vi "SiPM_Data_Analysis.vi"() -> ()   [LabVIEW 2019]
uses:
  <vilib>/Utility/tdmsutil.llb/fileViewerConfigData.ctl
  Data_Analysis_subvis/ESA_Data_Analysis_Global_VIs.vi
panel:
  in  "Detailed":bool
  out "Indicator":bool
  in  "Listbox":i32[](listbox) caption="SiPM_laser_tests_10x.tdms"
  in  "Data tab":enum32{"Raw", "Filtered", "Properties"}(tab)
  in  "Nb of Samples as Offset":i32=50
  in  "Display sel":bool
  out "SiPM Waveform":waveform(dbl)[](graph)
  in  "Nb of Samples to Display":i32=50
  in  "Tab Sel":T1(radio)
  out "Table":string[][](table)
  in  "Stop Button":bool
  in  "Open Button":bool
  out "Nb of Channels in Group":i32
  out "group names":string[](array[string])
  out "tdms file out":refnum<k34>
  in  "File contents":string[](tree)
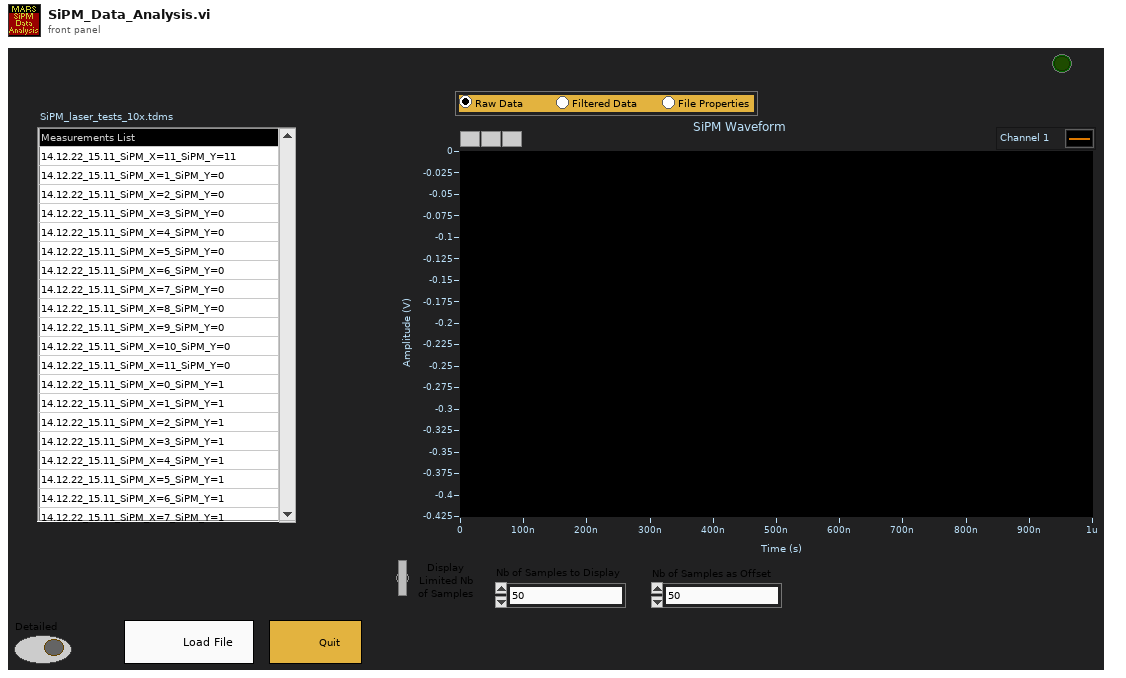
[diagram p1: front panel]
types:
  T1 = enum32{"Radio Selection 1", "Radio Selection 2", "Radio Selection 3"}
  T2 = typedef "fileViewerConfigData.ctl" = cluster{"Show all (table)":bool, "Show all (graph)":bool, "limit (table)":u64, "limit (graph)":u64, "no show":bool, "start (table)":u64, "start (graph)":u64}
  T3 = enum16{"open", "open or create", "create or replace", "create", "open (read-only)"}
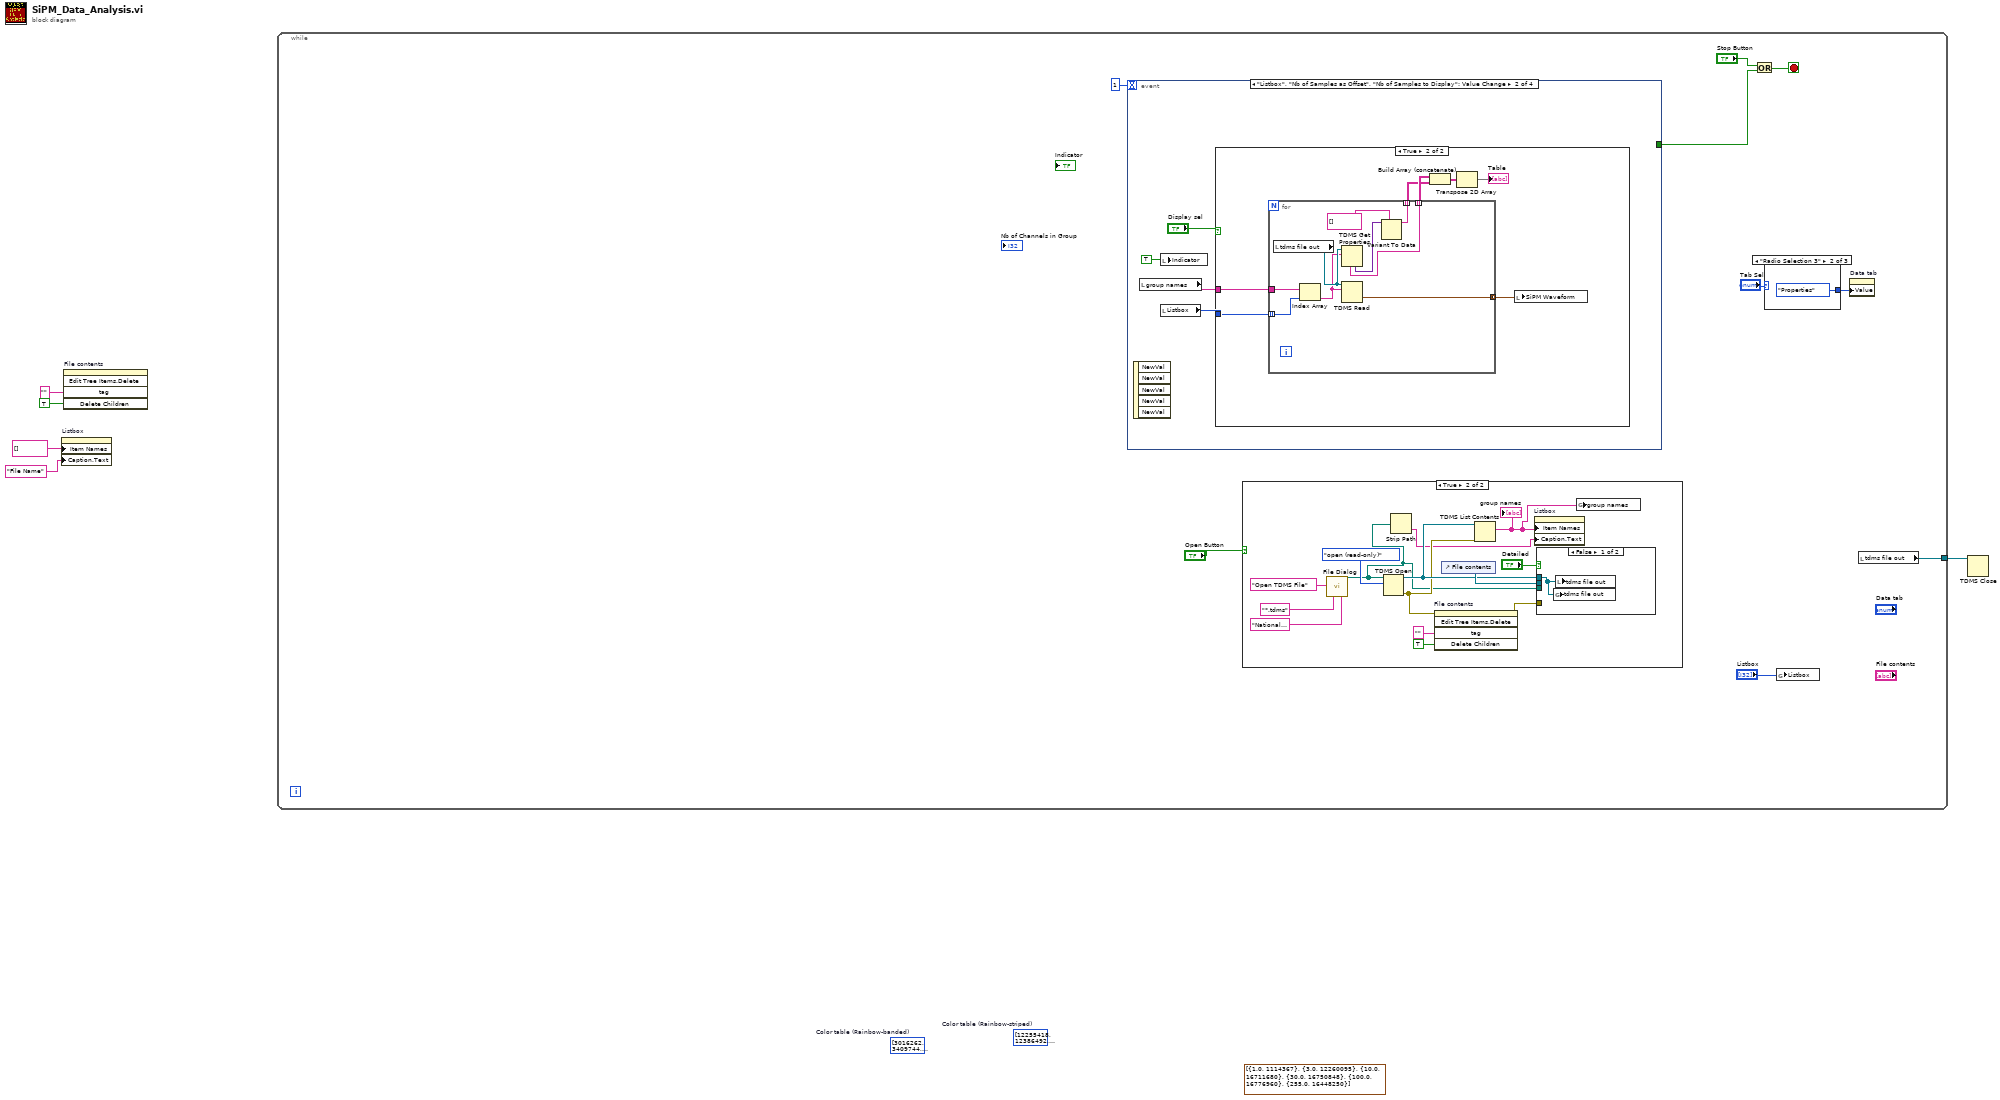
[diagram p0: block diagram]
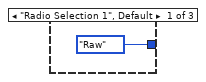
[diagram p2: hidden frame]
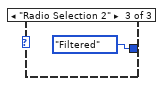
[diagram p3: hidden frame]
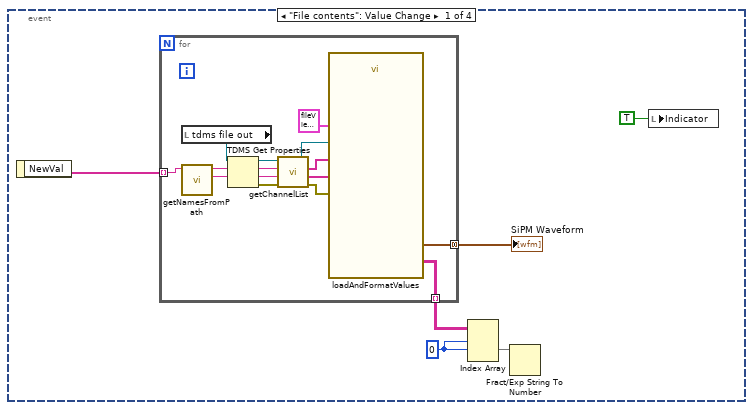
[diagram p4: hidden frame]
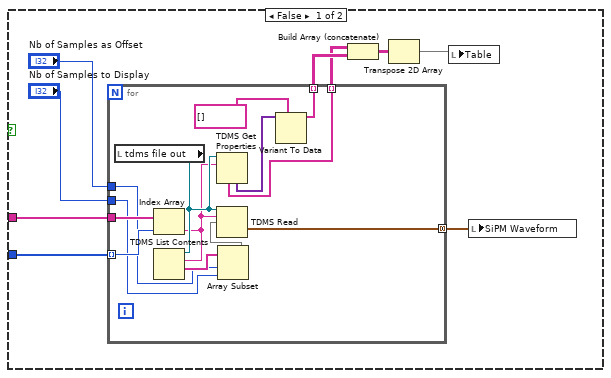
[diagram p5: hidden frame]
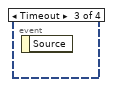
[diagram p6: hidden frame]
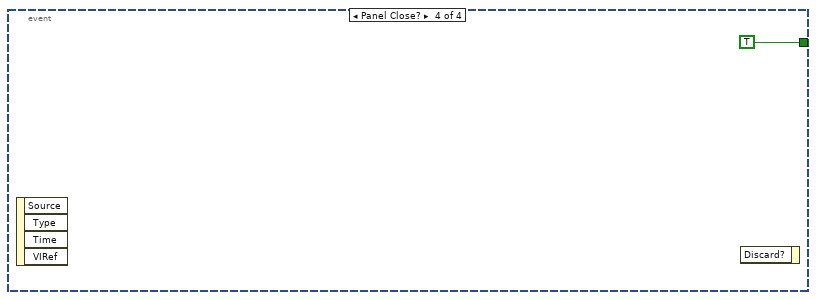
[diagram p7: hidden frame]
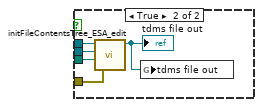
[diagram p9: hidden frame]
diagram:
  (unwired) cluster{dbl, u32}[] [{1.0, 1114367}, {3.0, 12260095}, {10.0, 16711680}, {30.0, 16750848}, {100.0, 16776960}, {255.0, 16448250}] ("Z Scale.Marker Values[]")
  (unwired) u32[] [12255418, 12386492, 12517567, 12320960, 12189888, 12058817, 11927746, 11731139, 11600067, 9175197, 9044125, 11141318, 11010246, 10813639, 10682568, 10551497, 10354890, 10223818, 10092747, 7930019, 7798948, 9633997, 9502926, 9306319, 9175248, 9044176, 8847569, 8716498, 8585427, 6750377, 6619306, 8126677, 7995606, 7798999, 7667927, 7536856, 7340249, 7209178, 7078106, 5505199, 5374128, 6619357, 6488285, 6291678, 6160607, 6029536, 5832929, 5701857, 5570786, 4325557, 4194486, 5112036, 4980965, 4784358, 4653287, 4522215, 4325608, 4194537, 4063466, 3080380, 3014844, 3604716, 3408109, 3277038, 3277038, 3145966, 3014895, 2818288, 2687217, 2556145, 1900738, 1769666, 2097396, 1900789, 1769717, 1638646, 1507575, 1310968, 1179896, 1048825, 721096, 590024, 590075, 393468, 262397, 131326, 255, 1791, 3327, 4863, 5068, 6348, 9471, 11007, 12543, 14079, 15615, 17151, 18687, 20223, 17612, 18636, 25087, 26623, 28159, 29695, 31231, 32767, 34303, 35839, 29900, 31180, 40447, 41983, 43775, 45311, 46847, 48383, 49919, 51455, 42444, 43724, 56063, 57599, 59135, 60671, 62207, 63743, 65535, 65528, 52418, 52413, 65510, 65504, 65498, 65492, 65486, 65480, 65474, 65468, 52369, 52364, 65449, 65443, 65437, 65431, 65425, 65419, 65413, 65407, 52321, 52316, 65389, 65383, 65377, 65371, 65364, 65358, 65352, 65346, 52272, 52267, 65328, 65322, 65316, 65310, 65304, 65298, 65292, 65286, 52224, 314368, 851712, 1244928, 1638144, 2031360, 2424576, 2817792, 3211008, 3604224, 3197952, 3525632, 4783872, 5177088, 5635840, 6029056, 6422272, 6815488, 7208704, 7601920, 6409216, 6736896, 6736896, 8781568, 9174784, 9568000, 9961216, 10354432, 10747648, 11206400, 11599616, 9554944, 9882624, 12779264, 13172480, 13565696, 13958912, 14352128, 14745344, 15138560, 15531776, 12766208, 13093888, 16776960, 16775170, 16773637, 16771847, 16770314, 16768780, 16766991, 16765457, 13411088, 13409810, 16760601, 16758812, 16757278, 16755745, 16753955, 16752422, 16750888, 16749099, 13398052, 13396774, 16744243, 16742704, 16741166, 16739884, 16738345, 16736807, 16735269, 16733730, 13385753, 13384728, 16729371, 16727833, 16726295, 16725012, 16723474, 16721936, 16720397, 16718859, 13373959, 13372677, 16714500, 16712962, 16711680]  # Color table (Rainbow-striped)
  (unwired) u32[] [3016262, 3409744, 4000097, 4721526, 5508493, 6229924, 6820281, 7214025, 7345364, 7279831, 6886611, 6362057, 5640632, 4788132, 4001165, 3214197, 2492769, 2033488, 1640006, 1508930, 1508934, 1640272, 1902945, 2165622, 2428301, 2690980, 2822585, 2888649, 2757844, 2626775, 2299091, 1971145, 1642936, 1249188, 920973, 724086, 592737, 461392, 395846, 396098, 396358, 462928, 595297, 727925, 861069, 994212, 1127608, 1260745, 1328083, 1329111, 1329876, 1264073, 1132217, 999844, 866957, 734070, 600929, 468304, 401734, 401730, 402502, 469584, 603489, 737909, 737909, 872845, 1008036, 1143224, 1277641, 1345747, 1347287, 1347796, 1281225, 1147833, 1013668, 878989, 743798, 609121, 475216, 407878, 407362, 408390, 476496, 611681, 747893, 884877, 1022116, 1158840, 1294793, 1363667, 1365719, 1365202, 1296836, 1161649, 1025178, 888194, 751211, 614742, 479302, 411196, 410168, 411193, 479297, 614732, 750939, 888171, 1025145, 1161350, 1296782, 1364883, 1365906, 1365132, 1296769, 1161588, 1025124, 888147, 751172, 614710, 479276, 411173, 410146, 411170, 479270, 614700, 750900, 888124, 1025091, 1161289, 1296716, 1364813, 1365834, 1365062, 1296703, 1161527, 1025070, 888101, 751133, 614678, 479249, 411149, 410124, 411147, 479244, 614668, 750861, 888078, 1156111, 1488913, 1820947, 2151188, 2414356, 2610196, 2738451, 2668817, 2597903, 2329869, 2061835, 1794313, 1593351, 1459718, 1458694, 1590790, 1921031, 2449673, 3110155, 3902733, 4695055, 5486609, 6211859, 6738708, 7132948, 7197716, 7063827, 6666513, 6136847, 5410061, 4617739, 3957001, 3362823, 2967046, 2900486, 3098118, 3690503, 4546825, 5666059, 6917389, 8233999, 9484305, 10537235, 11326228, 11786004, 11785236, 11785236, 11454739, 10729745, 9675791, 8424717, 7173643, 6054153, 5066759, 4474374, 4342278, 4605190, 5262855, 6380553, 7695883, 9273613, 10785807, 12100625, 13217555, 13874452, 14136340, 13938196, 13214227, 12161553, 10780431, 9267725, 7755531, 6374921, 5257479, 4599814, 4336646, 4599302, 5255943, 6372361, 7685899, 9261837, 10771983, 12085009, 13200659, 13856532, 14118164, 13920276, 13197075, 12145937, 10766351, 9255949, 7745547, 6366729, 5250567, 4593926, 4331014, 4593158, 5249287, 6364169, 7675915, 9249805, 10758159, 12069393, 13183507, 13838612, 14099988, 13902356, 13180179, 12130065, 10752527]  # Color table (Rainbow-banded)
  n1 = property on="Listbox" class="LstBox (strict)"("Item Names"=string[] [], "Caption.Text"="File Name") -> ()  [unwired: 2 in, 2 out]
  n2 = invoke on="File contents" class="Tree (strict)" method="Edit Tree Items.Delete"("tag"="" ("Tag"), "Delete Children"=TRUE ("Delete Children?")) -> ()  [unwired: 3 in, 5 out]
  n3 = while {
    tunnel: [w12] -> w5
    stop <- w9 stop-if-true
    n4 = event shown="[1] \"Listbox\", \"Nb of Samples as Offset\", \"Nb of Samples to Display\": Value Change" {
      selector: _ -> [_ _ _ _]
      dyn-events: _ -> [_ _ _ _]
      timeout: 1 -> [_ _ _ _]
      tunnel: [_ _ _ TRUE ("Stop Button")] -> w8
      event "File contents": Value Change {
        w20 = 0 ("disabled index (col)")
        n5 = event-data() -> ("NewVal"=w23:string[])  [unwired: 1 in]
        n6 = for {
          tunnel: [w25] -> w22 mode=concatenating
          tunnel: w23 -> [w26] mode=indexing
          tunnel: [w24] -> w21 mode=indexing
          n7 = local read "tdms file out"() -> (w32:refnum<k34>)
          n8 = call <vilib>:"getNamesFromPath.vi"("tree path"=w26) -> ("channel"=w33:string, "group"=w34:string)  [unwired: 1 in, 4 out]
          n9 = TDMS Get Properties(9:w33, 10:w34, 11:w32) -> (0:w37:errorcluster, 1:w36:string, 2:w35:string, 3:w38:refnum<k34>)  [unwired: 1 in, 4 out]
          n10 = call <vilib>:"getChannelList.vi"("error in (no error)"=w37, "channel names"=w36, "group name"=w35, "tdms file"=w38) -> ("error out"=w29:errorcluster, "channel names out"=w30:string[], "group names out"=w31:string[], "tdms file out"=w28:refnum<k34>)
          n11 = call <vilib>:"loadAndFormatValues.vi"("error in (no error)"=w29, "configuration"=T2 {"Show all (table)"=TRUE, "Show all (graph)"=TRUE, "limit (table)"=0, "limit (graph)"=0, "no show"=FALSE, "start (table)"=0, "start (graph)"=0}, "channel names"=w30, "group names"=w31, "tdms file"=w28) -> ("waveform values"=w25:waveform(dbl)[], "table values"=w24:string[][])  [unwired: 5 out]
        }
        "SiPM Waveform" <- w22
        n12 = Index Array(array=w21, index (dim 0)=w20, index (dim 1)=w20) -> (element=w19:string[])  [unwired: 1 in]
        n13 = Fract/Exp String To Number(string=w19) -> ()  [unwired: 3 in, 2 out]
        n14 = local write "Indicator"(TRUE ("Indicator")) -> ()
      }
      event "Listbox", "Nb of Samples as Offset", "Nb of Samples to Display": Value Change {
        n15 = event-data() -> ()  [unwired: 1 in, 5 out]
        n16 = local read "group names"() -> (w42:string[])
        n17 = local read "Listbox"() -> (w41:i32[])
        n18 = local write "Indicator"(TRUE ("Indicator")) -> ()
        n19 = case shown="True" "Display sel" {
          tunnel: w42 -> [w51 w71]
          tunnel: w41 -> [w50 w70]
          frame False {
            n20 = for {
              tunnel: w51 -> [w64]
              tunnel: w50 -> [w63] mode=indexing
              tunnel: [w52] -> w49 mode=concatenating
              tunnel: [w62] -> w46 mode=indexing
              tunnel: [w60] -> w47 mode=indexing
              tunnel: "Nb of Samples to Display" -> [w55]
              tunnel: "Nb of Samples as Offset" -> [w53]
              n21 = local read "tdms file out"() -> (w58:refnum<k34>)
              n22 = Index Array(array=w64, index=w63) -> (element=w57:string)
              n23 = TDMS List Contents(6:w57, 7:w58) -> (1:w56:string[])  [unwired: 1 in, 3 out]
              n24 = TDMS Get Properties(10:w57, 11:w58) -> (4:w59:variant[], 6:w62:string[])  [unwired: 4 in, 4 out]
              n25 = Array Subset(array=w56, index=w53, length=w55) -> (w54:string[])
              n26 = TDMS Read(0:w58, 5:w57, 7:w54) -> (10:w52:waveform(dbl)[])  [unwired: 5 in, 5 out]
              n27 = Variant To Data(type=string[] [] ("property names"), Variant=w59) -> (data=w60:string[])  [unwired: 1 in, 1 out]
            }
            n28 = Build Array (concatenate)(w46, w47) -> (w48:string[][])
            n29 = Transpose 2D Array(2D array=w48) -> (transposed array=w43:string[][])
            n30 = local write "Table"(w43) -> ()
            n31 = local write "SiPM Waveform"(w49) -> ()
          }
          frame True {
            n32 = for {
              tunnel: w71 -> [w80]
              tunnel: w70 -> [w79] mode=indexing
              tunnel: [w72] -> w65 mode=concatenating
              tunnel: [w76] -> w67 mode=indexing
              tunnel: [w74] -> w66 mode=indexing
              n33 = local read "tdms file out"() -> (w78:refnum<k34>)
              n34 = Index Array(array=w80, index=w79) -> (element=w77:string)
              n35 = TDMS Get Properties(10:w77, 11:w78) -> (4:w73:variant[], 6:w76:string[])  [unwired: 4 in, 4 out]
              n36 = TDMS Read(0:w78, 5:w77) -> (10:w72:waveform(dbl)[])  [unwired: 6 in, 5 out]
              n37 = Variant To Data(type=string[] [] ("property names"), Variant=w73) -> (data=w74:string[])  [unwired: 1 in, 1 out]
            }
            n38 = Build Array (concatenate)(w67, w66) -> (w69:string[][])
            n39 = Transpose 2D Array(2D array=w69) -> (transposed array=→"Table":string[][])
            n40 = local write "SiPM Waveform"(w65) -> ()
          }
        }
      }
      event Timeout {
        n41 = event-data() -> ()  [unwired: 1 in, 1 out]
      }
      event Panel Close? {
        n42 = event-data() -> ()  [unwired: 1 in, 4 out]
        n43 = event-data() -> ()  [unwired: 2 in, 1 out]
      }
    }
    n44 = case shown="True" "Open Button" {
      frame False {
      }
      frame True {
        n45 = call "File Dialog"("prompt"="Open TDMS File" ("prompt tdms"), "pattern (all files)"="*.tdms", "pattern label"="National Instruments TDM Streaming" ("pattern label tdms")) -> ("selected path"=w85:path)  [unwired: 4 in, 8 out]
        n46 = TDMS Open(10:T3."open (read-only)" ("operation (0:open)"), 11:w85) -> (0:w86:errorcluster, 3:w87:refnum<k34>)  [unwired: 5 in]
        n47 = Strip Path(path=w85) -> (name=w84:string)  [unwired: 1 out]
        n48 = invoke on="File contents" class="Tree (strict)" method="Edit Tree Items.Delete"(error in=w86, "tag"="" ("Tag"), "Delete Children"=TRUE ("Delete Children?")) -> (error out=w94:errorcluster)  [unwired: 2 in, 4 out]
        n49 = control-ref of="File contents"() -> (w95:refnum<vi>)
        n50 = TDMS List Contents(4:w86, 7:w87) -> (2:w83:string[])  [unwired: 1 in, 3 out]
        "group names" <- w83
        n51 = property on="Listbox" class="LstBox (strict)"("Item Names"=w83, "Caption.Text"=w84) -> ()  [unwired: 2 in, 2 out]
        n52 = case shown="False" "Detailed" {
          tunnel: w95 -> [_ w101]
          tunnel: w94 -> [_ w100]
          tunnel: w85 -> [_ w99]
          tunnel: w87 -> [w96 w98]
          frame False {
            n53 = global write "ESA_Data_Analysis_Global_VIs.vi" "tdms file out"(w96) -> ()
            n54 = local write "tdms file out"(w96) -> ()
          }
          frame True {
            n55 = call "initFileContentsTree_ESA_edit.vi"("error in (no error)"=w100, "file path"=w99, "Tree Refnum"=w101, "tdms file"=w98) -> ("tdms file out"=w97:refnum<k34>)  [unwired: 2 in, 1 out]
            "tdms file out" <- w97
            n56 = global write "ESA_Data_Analysis_Global_VIs.vi" "tdms file out"(w97) -> ()
          }
        }
        n57 = global write "ESA_Data_Analysis_Global_VIs.vi" "group names"(w83) -> ()
      }
    }
    n58 = Or(x="Stop Button", y=w8) -> (x .or. y?=w9:bool)
    n59 = case shown="\"Radio Selection 3\"" "Tab Sel" {
      tunnel: [enum32{"Raw", "Filtered", "Properties"}."Raw" ("Raw data") enum32{"Raw", "Filtered", "Properties"}."Properties" ("Raw data") enum32{"Raw", "Filtered", "Properties"}."Filtered" ("Raw data")] -> w10
      frame "Radio Selection 1", Default {
      }
      frame "Radio Selection 3" {
      }
      frame "Radio Selection 2" {
      }
    }
    n60 = global write "ESA_Data_Analysis_Global_VIs.vi" "Listbox"("Listbox") -> ()
    n61 = property on="Data tab" class="TabCtl (strict)"("Value"=w10) -> ()  [unwired: 2 in, 2 out]
    n62 = local read "tdms file out"() -> (w12:refnum<k34>)
  }
  n63 = TDMS Close(11:w5) -> ()  [unwired: 1 in, 2 out]
